vi "Projecte X.vi"() -> ()   [LabVIEW 2017]
uses:
  <vilib>/MakerHub/LINX/Public/Peripherals/PWM/PWM Set Duty Cycle 1 Chan.vi
  <vilib>/MakerHub/LINX/Public/Peripherals/Analog/Analog Read 1 Chan.vi
  <vilib>/MakerHub/LINX/Public/Peripherals/Analog/Analog Read N Chans.vi
  <vilib>/MakerHub/LINX/Private/Local IO/LinxAnalogRead.vi
  <vilib>/MakerHub/LINX/Public/Utilities/Check Channel.vi
  <vilib>/MakerHub/LINX/Public/Utilities/Open Serial.vi
  <vilib>/MakerHub/LINX/Public/Peripherals/PWM/PWM Set Duty Cycle N Chans.vi
  <vilib>/MakerHub/LINX/Private/Utilties/Generate Error.vi
  <vilib>/MakerHub/LINX/LMH-LINX.lvlib
panel:
  out "?":dbl(knob) scale=0.0..150.0
  out "Error Fitxer":errorcluster
  in  "Accés (0:read/write)":enum16{"read/write", "read-only", "write-only"}(ring)
  in  "Operació (0:open)":T1(ring)
  in  "Fitxer":path
  out "Velocitat (cm/s)":dbl
  out "Temps (s)":dbl
  in  "Distància entre referències":dbl
  out "Dades de les franges":u32[](array[numeric])
  out "Temps instantani":u32
  out "Dades completes":u32[](array[numeric])
  in  "A llindar":dbl
  out "Intensitat vs Temps (instantani)":dbl(graph)
  out "B":u8
  out "R":u8
  out "G":u8
  out "Error RGB":errorcluster
  in  "Color":u32(colorbox)
  out "Intenstiat vs temps":cluster{"Y":dbl[], "Y":dbl[]}[](graph)
  in  "Stop":bool caption="STOP"
  in  "Serial Port":refnum<visa-resource-name>="N/A"
  in  "Analog Channel":u8
  out "Error Sensor":errorcluster
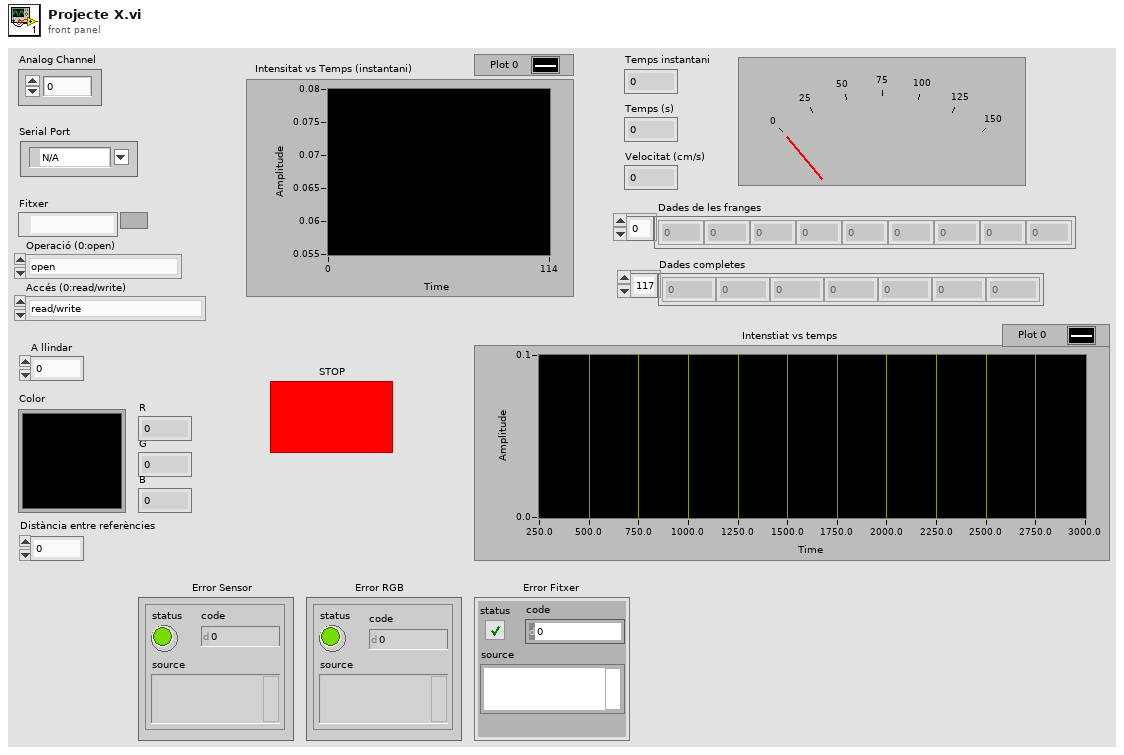
[diagram p1: front panel]
types:
  T1 = enum16{"open", "replace", "create", "open or create", "replace or create", "replace or create with confirmation"}
  T2 = typedef "LMH-LINX.lvlib/LINX Ref.ctl" = cluster{"IO":T3, "Interface":T4, "LINX Device Config":T5}
  T3 = typedef "LMH-LINX.lvlib/Platform.ctl" = enum16{"Remote", "Local"}
  T4 = typedef "LMH-LINX.lvlib/Interface.ctl" = enum16{"Serial", "TCP"}
  T5 = typedef "LMH-LINX.lvlib/Device.lvlib/LINX Device Config.ctl" = cluster{"Interface":T4, "COM Port":refnum<visa-resource-name>, "TCP Configuration":T6, "Device Family":u8, "Device ID":u8, "Device Name":string, "TCP Ref":refnum<k5>, "Channels":T7}
  T6 = typedef "LMH-LINX.lvlib/Device.lvlib/TCP Config.ctl" = cluster{"IP Address":string, "Port":u16}
  T7 = typedef "LMH-LINX.lvlib/Channels.ctl" = cluster{"DI":u8[], "DO":u8[], "AI":u8[], "AO":u8[], "PWM":u8[], "QE":u8[], "UART":u8[], "I2C 2":u8[], "SPI":u8[], "CAN":u8[], "Servo":u8[], "AI Ref (V)":dbl, "AI Resolution (Bits)":u8, "AO Ref (V)":dbl, "AO Resolution (Bits)":u8}
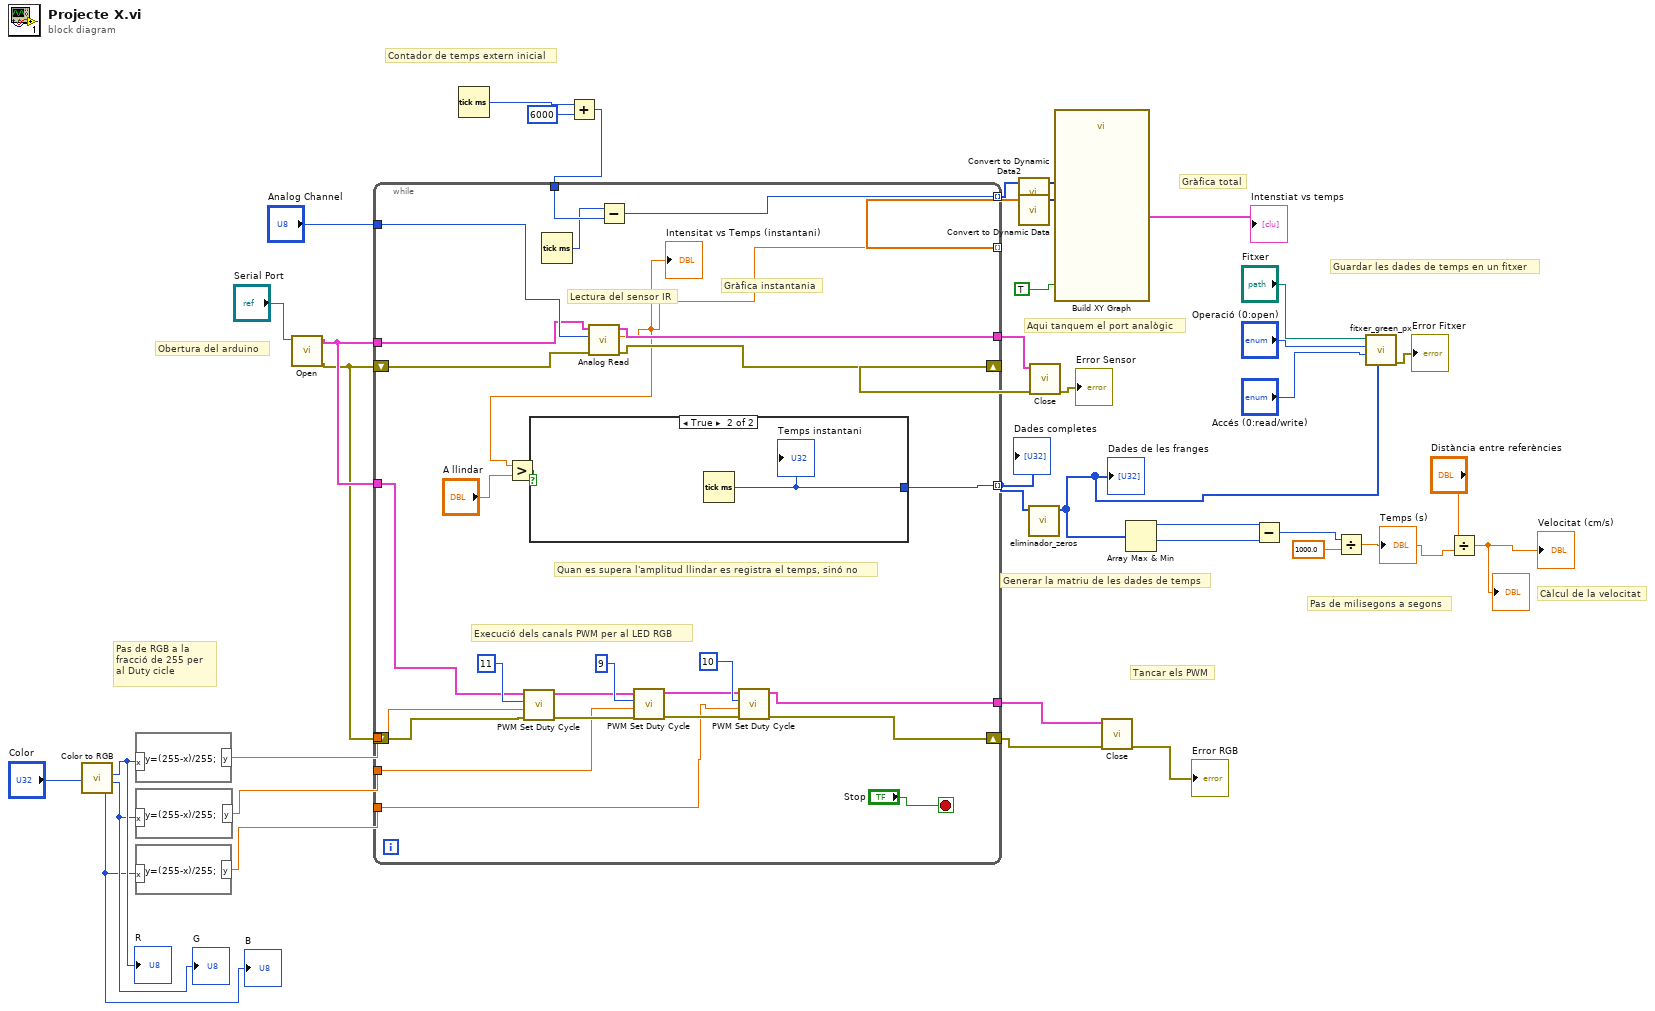
[diagram p0: block diagram]
diagram:
  # "Aqui tanquem el port analògic"
  # "Generar la matriu de les dades de temps"
  # "Guardar les dades de temps en un fitxer"
  # "Càlcul de la velocitat"
  # "Pas de milisegons a segons"
  # "Tancar els PWM"
  # "Gràfica total"
  # "Pas de RGB a la fracció de 255 per al Duty cicle"
  # "Obertura del arduino"
  # "Contador de temps extern inicial"
  n1 = call <vilib>:"Color to RGB.vi"("Color"="Color") -> ("R"=w21:u8, "G"=w20:u8, "B"=w19:u8)  [unwired: 1 out]
  "G" <- w20
  "R" <- w21
  "B" <- w19
  n2 = formula code="y=(255-x)/255;"("x"=w21) -> ("y"=w24:dbl)
  n3 = formula code="y=(255-x)/255;"("x"=w20) -> ("y"=w23:dbl)
  n4 = formula code="y=(255-x)/255;"("x"=w19) -> ("y"=w22:dbl)
  n5 = call-poly <vilib>:"Open.vi"("Serial Port"="Serial Port") -> ("Error Out"=w26:errorcluster, "LINX Resource"=w32:T2)  [unwired: 8 in, 1 out]
  n6 = Tick Count (ms)() -> (millisecond timer value=w18:u32)
  n7 = Add(x=w18, y=u32 6000) -> (x+y=w16:u32)
  n8 = while {
    tunnel: w32 -> [w62]
    tunnel: [w59] -> w28
    tunnel: "Analog Channel" -> [w63]
    shift-right: [w60] -> w29
    shift-left: w26 -> [w61]
    tunnel: [w45] -> w36 mode=indexing
    tunnel: w16 -> [w66]
    tunnel: [w64] -> w33 mode=indexing
    tunnel: w32 -> [w46]
    shift-right: [w40] -> w1
    shift-left: w26 -> [w53]
    tunnel: [w50] -> w25
    tunnel: w24 -> [w49]
    tunnel: w23 -> [w48]
    tunnel: w22 -> [w47]
    tunnel: [w41] -> w15 mode=indexing
    stop <- "Stop" stop-if-true
    # "Gràfica instantania"
    # "Quan es supera l'amplitud llindar es registra el temps, sinó no"
    # "Lectura del sensor IR"
    # "Execució dels canals PWM per al LED RGB"
    n9 = call-poly <vilib>:"PWM Set Duty Cycle.vi"("Error In"=w53, "Duty Cycle (0-1)"=w49, "PWM Channel"=u8 11, "LINX Resource"=w46) -> ("Error Out"=w52:errorcluster, "LINX Resource"=w55:T2)  [unwired: 6 in]
    n10 = Tick Count (ms)() -> (millisecond timer value=w65:u32)
    n11 = call-poly <vilib>:"Analog Read.vi"("Error In"=w61, "Analog Channel"=w63, "LINX Resource"=w62) -> ("Error Out"=w60:errorcluster, "Voltage"=w45:dbl, "LINX Resource"=w59:T2)  [unwired: 5 in, 1 out]
    "Intensitat vs Temps (instantani)" <- w45
    n12 = Greater?(x=w45, y="A llindar") -> (0:w42:bool)
    n13 = case shown="True" w42 {
      tunnel: [_ w67] -> w41
      frame False {
      }
      frame True {
        n14 = Tick Count (ms)() -> (millisecond timer value=w67:u32)
        "Temps instantani" <- w67
      }
    }
    n15 = Subtract(x=w65, y=w66) -> (x-y=w64:u32)
    n16 = call-poly <vilib>:"PWM Set Duty Cycle.vi"("Error In"=w52, "Duty Cycle (0-1)"=w48, "PWM Channel"=u8 9, "LINX Resource"=w55) -> ("Error Out"=w51:errorcluster, "LINX Resource"=w54:T2)  [unwired: 6 in]
    n17 = call-poly <vilib>:"PWM Set Duty Cycle.vi"("Error In"=w51, "Duty Cycle (0-1)"=w47, "PWM Channel"=u8 10, "LINX Resource"=w54) -> ("Error Out"=w40:errorcluster, "LINX Resource"=w50:T2)  [unwired: 6 in]
  }
  "Dades completes" <- w15
  n18 = call "Convert to Dynamic Data2"("Array"=w33) -> ("Dynamic Data Type"=w34:dynamicdata)  [unwired: 3 in]
  n19 = call "Convert to Dynamic Data"("Array"=w36) -> ("Dynamic Data Type"=w35:dynamicdata)  [unwired: 3 in]
  n20 = call "eliminador_zeros.vi"("Array in"=w15) -> ("Array out"=w7:u32[])  [unwired: 10 in]
  "Dades de les franges" <- w7
  n21 = call <vilib>:"Close.vi"("Error In"=w29, "LINX Resource"=w28) -> ("Error Out"=→"Error Sensor":errorcluster)  [unwired: 9 in]
  n22 = call "Build XY Graph"("Reset"=TRUE, "Y Input"=w35, "X Input"=w34) -> ("XY Graph"=→"Intenstiat vs temps":cluster{"X":dbl[], "Y":dbl[]}[])  [unwired: 7 in, 1 out]
  n23 = call <vilib>:"Close.vi"("Error In"=w1, "LINX Resource"=w25) -> ("Error Out"=→"Error RGB":errorcluster)  [unwired: 9 in]
  n24 = Array Max & Min(array=w7) -> (max value=w14:u32, min value=w13:u32)  [unwired: 2 out]
  n25 = Subtract(x=w14, y=w13) -> (x-y=w10:u32)
  n26 = Divide(x=w10, y=1000.0) -> (x/y=w9:dbl)
  "Temps (s)" <- w9
  n27 = call "fitxer_green_px.vi"("Array in"=w7, "access (0:read/write)"="Accés (0:read/write)", "operation (0:open)"="Operació (0:open)", "file path (use dialog)"="Fitxer") -> ("error out"=→"Error Fitxer":errorcluster)  [unwired: 7 in]
  n28 = Divide(x="Distància entre referències", y=w9) -> (x/y=→"Velocitat (cm/s)" →"?":dbl)
